vi "CreatePen.vi"(8 "error in (no error)":errorcluster, 10 "Pen(Width=1, Solid)":T1, 11 "ColorRef":refnum<k24>) -> (0 "error out":errorcluster, 3 "PenRef":refnum<k24>)   [LabVIEW 2020, in "LcPictureBox.lvclass"]
uses:
  LcPictureBox.lvclass
  System.Drawing
  Pen.ctl
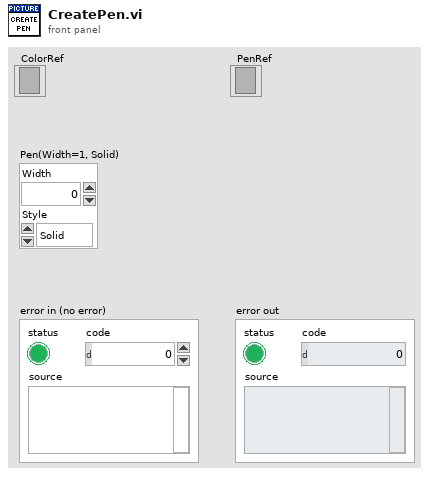
[diagram p1: front panel]
types:
  T1 = typedef "LcPictureBox.lvclass/Pen.ctl" = cluster{"Width":u16, "Style":enum32{"Solid", "Dash", "Dot", "DashDot", "DashDotDot"}}
  T2 = enum32{"Solid", "Dash", "Dot", "DashDot", "DashDotDot"}
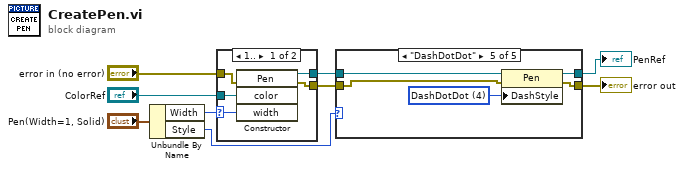
[diagram p0: block diagram]
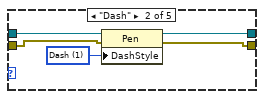
[diagram p3: hidden frame]
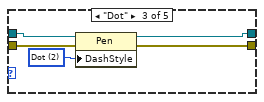
[diagram p4: hidden frame]
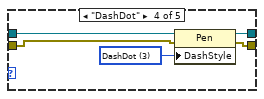
[diagram p5: hidden frame]
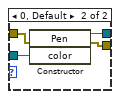
[diagram p6: hidden frame]
diagram:
  n1 = Unbundle By Name("Pen(Width=1, Solid)") -> ("Width"=w9:u16, "Style"=w5:T2)
  n2 = case shown="1.." w9 {
    selector: w9 -> [w12 _]
    tunnel: [w14 w18] -> w3
    tunnel: [w13 w17] -> w4
    tunnel: "error in (no error)" -> [w11 w16]
    tunnel: "ColorRef" -> [w10 w15]
    frame 1.. {
      n3 = constructor class="Pen"(error in=w11, "color"=w10, "width"=w12) -> (reference out=w14:refnum<k24>, error out=w13:errorcluster)  [unwired: 2 in, 3 out]
    }
    frame 0, Default {
      n4 = constructor class="Pen"(error in=w16, "color"=w15) -> (reference out=w18:refnum<k24>, error out=w17:errorcluster)  [unwired: 2 in, 2 out]
    }
  }
  n5 = case shown="\"DashDotDot\"" w5 {
    tunnel: w4 -> [w19 w25 w30 w35 w40]
    tunnel: w3 -> [w20 w24 w29 w34 w39]
    tunnel: [w20 w21 w26 w31 w36] -> w1
    tunnel: [w19 w22 w27 w32 w37] -> w2
    frame "Solid", Default {
    }
    frame "Dash" {
      w23 = 1 items=["Solid", "Dash", "Dot", "DashDot", "DashDotDot", "Custom"] ("DashStyle")
      n6 = property class="Pen"(reference=w24, error in=w25, "DashStyle"=w23) -> (reference out=w21:refnum<k24>, error out=w22:errorcluster)
    }
    frame "Dot" {
      w28 = 2 items=["Solid", "Dash", "Dot", "DashDot", "DashDotDot", "Custom"] ("DashStyle")
      n7 = property class="Pen"(reference=w29, error in=w30, "DashStyle"=w28) -> (reference out=w26:refnum<k24>, error out=w27:errorcluster)
    }
    frame "DashDot" {
      w33 = 3 items=["Solid", "Dash", "Dot", "DashDot", "DashDotDot", "Custom"] ("DashStyle")
      n8 = property class="Pen"(reference=w34, error in=w35, "DashStyle"=w33) -> (reference out=w31:refnum<k24>, error out=w32:errorcluster)
    }
    frame "DashDotDot" {
      w38 = 4 items=["Solid", "Dash", "Dot", "DashDot", "DashDotDot", "Custom"] ("DashStyle")
      n9 = property class="Pen"(reference=w39, error in=w40, "DashStyle"=w38) -> (reference out=w36:refnum<k24>, error out=w37:errorcluster)
    }
  }
  "PenRef" <- w1
  "error out" <- w2
